vi "Insight_Measure_FFT_Window.vi"(8 "error in (no error)":errorcluster, 9 "Mode (Read / Write)":enum8{"Write", "Read"}(ring), 10 "Window":T1=enum."Hamming", 11 "telnet connection":T2) -> (0 "error out":errorcluster, 1 "Window?":T1=enum."Hamming", 2 "response data":string, 3 "telnet  connection out":T2)   [LabVIEW 2011]
doc: "Insight Photonic Solutions\n\nThis VI sets the Window used to calculate the FFT in Measurement Mode.\n\nver 1.0 - original release\nver 3.2 - make Enum for windows the same as Update_PSF.vi, for easier integration of both into programs. Also, added parsing for command versions before and after Atlas version 3.2\nver 3.3 - modify internal parser to recognize all 4 letters of window options capitalized."
uses:
  Telnet Session.ctl
  Window_Functions.ctl
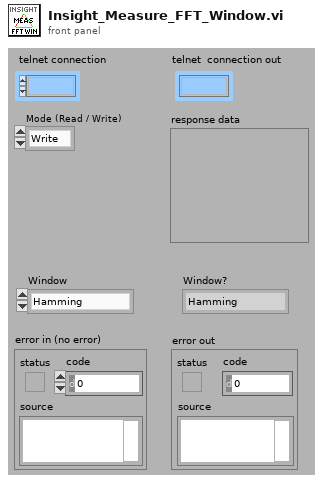
[diagram p1: front panel]
types:
  T1 = typedef "Window_Functions.ctl" = enum16{"Rectangular", "Hann", "Hamming", "Blackman", "Blackman-Harris"}
  T2 = typedef "Telnet Session.ctl" = refnum<k1>
  T3 = enum16{"RECTangular", "HANN", "HAMMing", "BLACkman", "BHARris"}
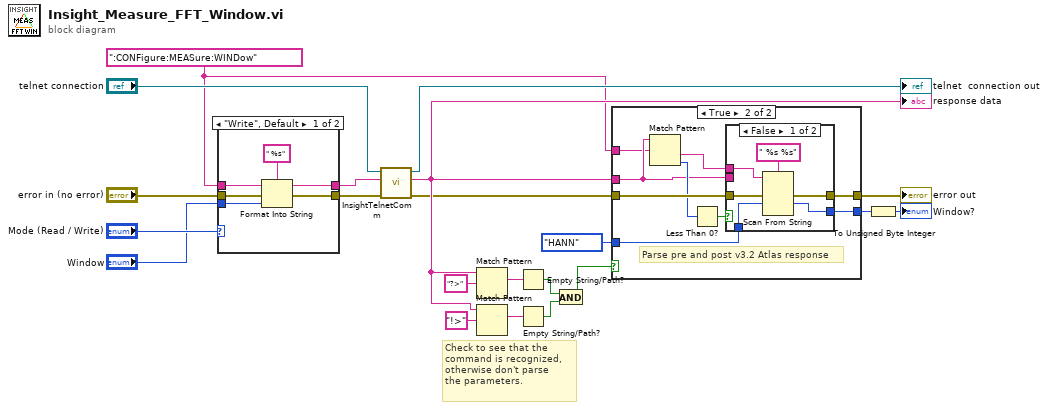
[diagram p0: block diagram]
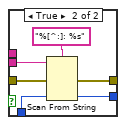
[diagram p3: hidden frame]
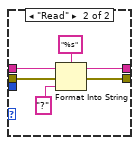
[diagram p4: hidden frame]
diagram:
  w2 = ":CONFigure:MEASure:WINDow" ("String")
  # "Check to see that the \ncommand is recognized,\notherwise don't parse \nthe parameters."
  n1 = case shown="\"Write\", Default" "Mode (Read / Write)" {
    tunnel: [w27 w29] -> w19
    tunnel: "error in (no error)" -> [w26 w28]
    tunnel: w2 -> [w25 w31]
    tunnel: "Window" -> [w24 _]
    tunnel: [w22 w30] -> w18
    frame "Write", Default {
      n2 = Format Into String(format string=" %s", initial string=w25, error in=w26, w24) -> (resulting string=w22:string, error out=w27:errorcluster)
    }
    frame "Read" {
      n3 = Format Into String(format string="%s", initial string=w31, error in=w28, "?" ("input 1")) -> (resulting string=w30:string, error out=w29:errorcluster)
    }
  }
  n4 = call "InsightTelnetComm.vi"("error in"=w19, "write buffer (\"\")"=w18, "telnet connection"="telnet connection") -> ("error out"=w7:errorcluster, "response data"=w8:string, "telnet  connection out"=→"telnet  connection out":T2)  [unwired: 4 in]
  "response data" <- w8
  n5 = Match Pattern(string=w8, regular expression="?>") -> (match substring=w14:string)  [unwired: 1 in, 3 out]
  n6 = Match Pattern(string=w8, regular expression="!>") -> (match substring=w13:string)  [unwired: 1 in, 3 out]
  n7 = Empty String/Path?(string/path=w14) -> (empty?=w11:bool)
  n8 = Empty String/Path?(string/path=w13) -> (empty?=w10:bool)
  n9 = And(x=w11, y=w10) -> (x .and. y?=w6:bool)
  n10 = case shown="True" w6 {
    tunnel: [w35 w42] -> w5
    tunnel: w7 -> [w35 w41]
    tunnel: w8 -> [_ w38]
    tunnel: [w34 w43] -> w3
    tunnel: w2 -> [_ w37]
    tunnel: T3."HANN" ("Window") -> [w34 w36]
    frame False {
    }
    frame True {
      # "Parse pre and post v3.2 Atlas response"
      n11 = Match Pattern(string=w38, regular expression=w37) -> (after substring=w39:string, offset past match=w40:i32)  [unwired: 1 in, 2 out]
      n12 = Less Than 0?(x=w40) -> (x < 0?=w44:bool)
      n13 = case shown="False" w44 {
        tunnel: w39 -> [w49 _]
        tunnel: w38 -> [_ w55]
        tunnel: [w50 w56] -> w42
        tunnel: [w47 w53] -> w43
        tunnel: w41 -> [w46 w52]
        tunnel: w36 -> [w45 w51]
        frame False {
          n14 = Scan From String(format string=" %s %s" ("f"), input string=w49, error in=w46, default 1=w45) -> (error out=w50:errorcluster, output 1=w47:T3)  [unwired: 3 in, 2 out]
        }
        frame True {
          n15 = Scan From String(format string="%[^:]: %s", input string=w55, error in=w52, default 2=w51) -> (error out=w56:errorcluster, output 2=w53:T3)  [unwired: 3 in, 2 out]
        }
      }
    }
  }
  "error out" <- w5
  n16 = To Unsigned Byte Integer(number=w3) -> (unsigned 8bit integer=→"Window?":u8)
